vi "remove last element_plots.vi"(11 "Input":cluster{cluster{dbl, "icn":dbl}[]}[](array[cluster])) -> (3 "subarray":cluster{cluster{dbl, "icn":dbl}[]}[](array[cluster]))   [LabVIEW 2023]
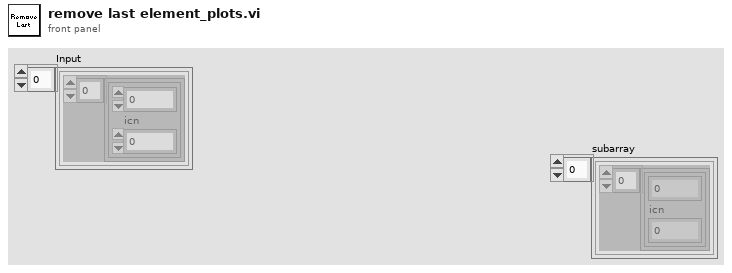
[diagram p1: front panel]
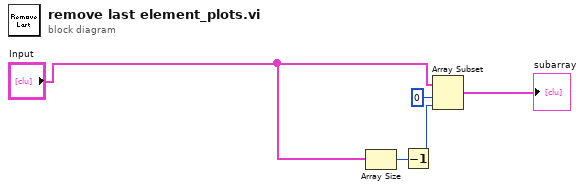
[diagram p0: block diagram]
diagram:
  n1 = Array Size(array="Input") -> (size(s)=w4:i32)
  n2 = Decrement(x=w4) -> (x-1=w3:i32)
  n3 = Array Subset(array="Input", index=0, length=w3) -> (→"subarray":cluster{cluster{dbl, "icn":dbl}[]}[])
